vi "pf_Get_3D-Data_Profile.vi"(6 "Mirror Profile? (F)":bool, 7 "Reverse Peak? (F)":bool, 8 "error in (no error)":errorcluster, 10 "Aquired Image":T1, 11 "IMAQ Session in":refnum<k11>) -> (0 "error out":errorcluster, 1 "Quality Profile":u8[](array[numeric]), 2 "Width Profile":sgl[](array[numeric]), 3 "IMAQ Session out":refnum<k11>, 5 "Peak Profile":sgl[](array[numeric]))   [LabVIEW 2025, in "Photonfocus_Toolkit.lvlib"]
doc: "Extracts profiles of 3D Data (Quality, Width and Peak) from an acquired image.\nPlease note that this function requires either a '2D and 3D mode' or '3D mode' set into the camera."
uses:
  Photonfocus_Toolkit.lvlib
  <vilib>/vision/Image Controls.llb/IMAQ Image.ctl
  _Private/Controls/pf_Camera_ctrl_mngr_action.ctl
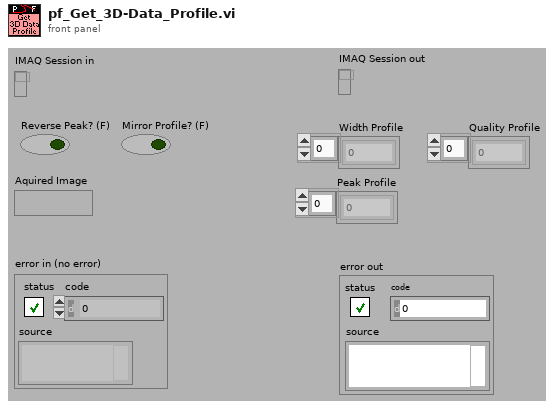
[diagram p1: front panel]
types:
  T1 = typedef "IMAQ Image.ctl" = refnum<image>
  T2 = typedef "Photonfocus_Toolkit.lvlib/pf_Camera_ctrl_mngr_action.ctl" = enum16{"Create", "Destroy", "Set", "Get"}
  T3 = typedef "Photonfocus_Toolkit.lvlib/pf_Camera_Control.ctl" = cluster{"Port Name":string, "Port Number":i32, "IMAQ Session":refnum<k11>, "PeakDetector_Mode":T4, "Window.W":u32, "Window.H":u32}
  T4 = typedef "Photonfocus_Toolkit.lvlib/pf_PeakDetector_Mode.ctl" = enum16{"Undefined", "2D only", "2D and 3D", "3D only"}
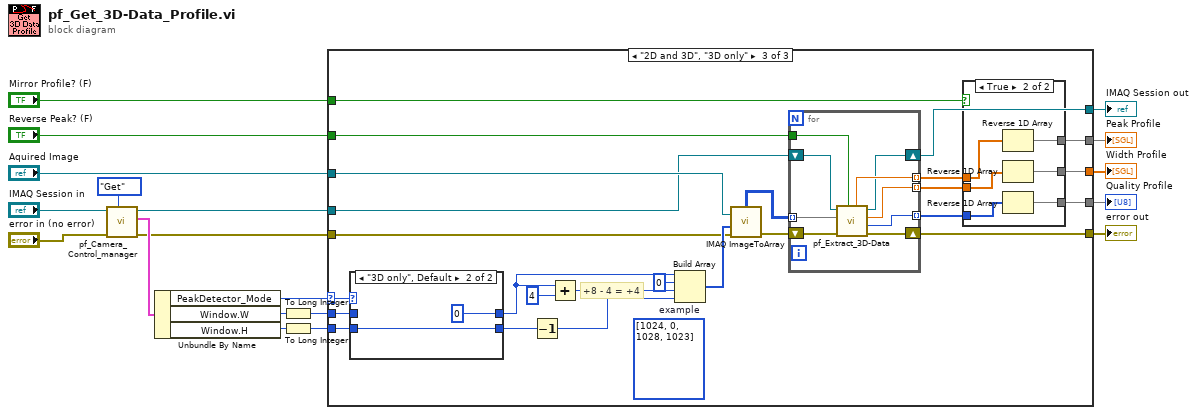
[diagram p0: block diagram]
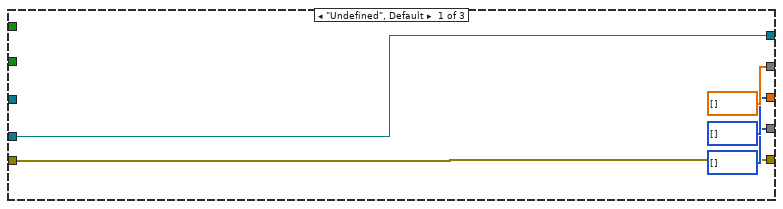
[diagram p2: hidden frame]
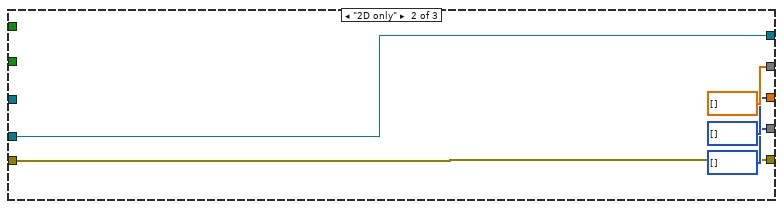
[diagram p3: hidden frame]
diagram:
  n1 = call "pf_Camera_Control_manager.vi"("Action"=pf_Camera_ctrl_mngr_action."Get", "error in (no error)"="error in (no error)", "IMAQ Session in"="IMAQ Session in") -> ("error out"=w6:errorcluster, "Camera Control out"=w10:T3, "IMAQ Session out"=w5:refnum<k11>)  [unwired: 1 in, 5 out]
  n2 = Unbundle By Name(w10) -> ("PeakDetector_Mode"=w4:T4, "Window.W"=w3:u32, "Window.H"=w8:u32)
  n3 = To Long Integer(number=w3) -> (32bit integer=w9:i32)
  n4 = To Long Integer(number=w8) -> (32bit integer=w7:i32)
  n5 = case shown="\"2D and 3D\", \"3D only\"" w4 {
    selector: w4 -> [_ _ w35]
    tunnel: "Aquired Image" -> [_ _ w54]
    tunnel: [sgl[] [] sgl[] [] w52] -> w18
    tunnel: [u8[] [] u8[] [] w50] -> w17
    tunnel: [u8[] [] u8[] [] w48] -> w16
    tunnel: [w24 w29 w47] -> w15
    tunnel: [w20 w25 w44] -> w14
    tunnel: w9 -> [_ _ w34]
    tunnel: w7 -> [_ _ w32]
    tunnel: w6 -> [w20 w25 w40]
    tunnel: w5 -> [w24 w29 w39]
    tunnel: "Reverse Peak? (F)" -> [_ _ w36]
    tunnel: "Mirror Profile? (F)" -> [_ _ w30]
    frame "Undefined", Default {
    }
    frame "2D only" {
    }
    frame "2D and 3D", "3D only" {
      (unwired) i32[] [1024, 0, 1028, 1023]  # example
      # "+8 - 4 = +4"
      n6 = case shown="\"3D only\", Default" w35 {
        tunnel: w34 -> [w65 _]
        tunnel: [w65 0] -> w33
        tunnel: w32 -> [w64 w66]
        tunnel: [w64 w66] -> w31
        frame "2D and 3D" {
        }
        frame "3D only", Default {
        }
      }
      n7 = Decrement(x=w31) -> (x-1=w38:i32)
      n8 = Add(x=w33, y=4) -> (x+y=w37:i32)
      n9 = Build Array(w33, 0, w37, w38) -> (w41:i32[])
      n10 = call "IMAQ ImageToArray"("error in (no error)"=w40, "Optional Rectangle"=w41, "Image"=w54) -> ("error out"=w46:errorcluster, "Image Pixels (U8)"=w45:u8[][])  [unwired: 4 out]
      n11 = for {
        shift-right: [w75] -> w44
        shift-left: w46 -> [w76]
        tunnel: [w72] -> w53 mode=indexing
        tunnel: w45 -> [w71] mode=indexing
        tunnel: [w74] -> w51 mode=indexing
        tunnel: [w73] -> w49 mode=indexing
        shift-right: [w69] -> w47
        shift-left: w39 -> [w70]
        tunnel: w36 -> [w68]
        n12 = call "pf_Extract_3D-Data.vi"("Reverse? (F)"=w68, "error in (no error)"=w76, "3D Data in"=w71, "IMAQ Session in"=w70) -> ("error out"=w75:errorcluster, "Quality out"=w73:u8, "Width out"=w74:sgl, "IMAQ Session out"=w69:refnum<k11>, "Peak out"=w72:sgl)  [unwired: 3 out]
      }
      n13 = case shown="True" w30 {
        tunnel: w53 -> [w57 w63]
        tunnel: [w57 w62] -> w52
        tunnel: w51 -> [w56 w61]
        tunnel: [w56 w60] -> w50
        tunnel: w49 -> [w55 w59]
        tunnel: [w55 w58] -> w48
        frame False {
        }
        frame True {
          n14 = Reverse 1D Array(array=w63) -> (reversed array=w62:sgl[])
          n15 = Reverse 1D Array(array=w61) -> (reversed array=w60:sgl[])
          n16 = Reverse 1D Array(array=w59) -> (reversed array=w58:u8[])
        }
      }
    }
  }
  "Peak Profile" <- w18
  "error out" <- w14
  "Width Profile" <- w17
  "Quality Profile" <- w16
  "IMAQ Session out" <- w15
